vi "limeDistance.vi"(11 "a2":dbl) -> (3 "d":dbl)   [LabVIEW 2019]
panel:
  in  "a1":dbl
  in  "h1":dbl
  in  "h2":dbl
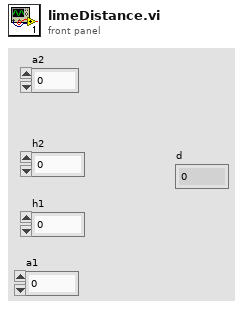
[diagram p1: front panel]
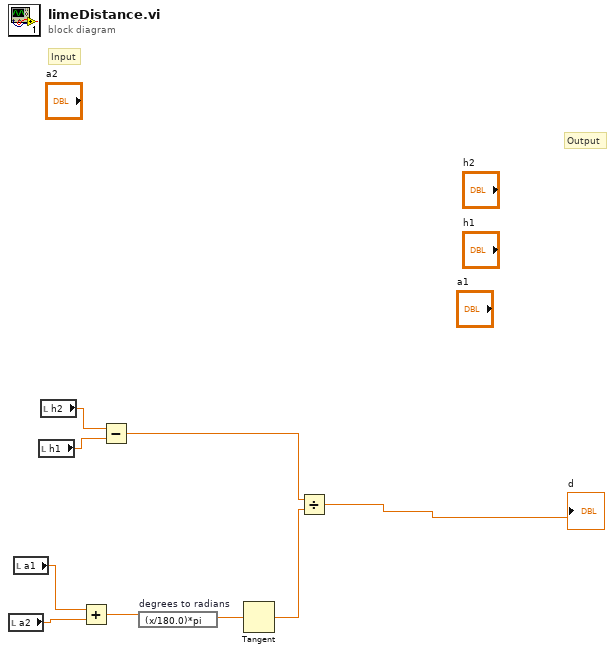
[diagram p0: block diagram]
diagram:
  # "Output"
  # "Input"
  n1 = local read "a2"() -> (w5:dbl)
  n2 = local read "a1"() -> (w6:dbl)
  n3 = local read "h1"() -> (w8:dbl)
  n4 = local read "h2"() -> (w9:dbl)
  n5 = Add(x=w6, y=w5) -> (x+y=w4:dbl)
  n6 = Subtract(x=w9, y=w8) -> (x-y=w3:dbl)
  n7 = expression code="(x/180.0)*pi" "degrees to radians"(w4) -> (w7:dbl)
  n8 = Tangent(1:w7) -> (0:w2:dbl)
  n9 = Divide(x=w3, y=w2) -> (x/y=→"d":dbl)
